vi "Snap to right (centered).vi"(1 "Large Rect":T1, 2 "Small Rect":T1) -> (0 "Snapped to right center":T1)   [LabVIEW 2012]
doc: "This VI calculates the position of a snapped-to-right rectangle from the positions of a large rectangle and a smaller one that will be positioned inside."
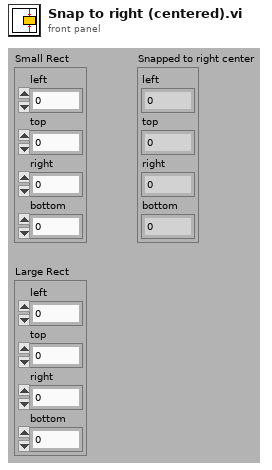
[diagram p1: front panel]
types:
  T1 = cluster{"left":i16, "top":i16, "right":i16, "bottom":i16}
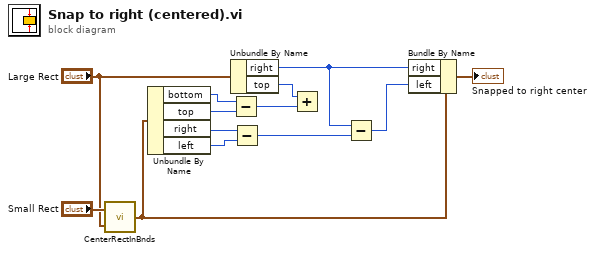
[diagram p0: block diagram]
diagram:
  n1 = call <vilib>:"CenterRectInBnds.vi"("bounds"="Large Rect", "rect"="Small Rect") -> ("centered rect"=w10:T1)
  n2 = Unbundle By Name(w10) -> ("bottom"=w13:i16, "top"=w12:i16, "right"=w5:i16, "left"=w4:i16)
  n3 = Unbundle By Name("Large Rect") -> ("right"=w3:i16, "top"=w9:i16)
  n4 = Subtract(x=w13, y=w12) -> (x-y=w11:i16)
  n5 = Subtract(x=w5, y=w4) -> (x-y=w2:i16)
  n6 = Add(x=w9, y=w11) -> ()  [unwired: 1 out]
  n7 = Subtract(x=w3, y=w2) -> (x-y=w1:i16)
  n8 = Bundle By Name(cluster=w10, "right"=w3, "left"=w1) -> (→"Snapped to right center":T1)
